vi "AddControlClass.vi"(4 "class":string, 5 "name":string, 6 "error in":errorcluster, 9 "PythonConverter_GUI in":refnum<class "PythonConverter_GUI.lvclass">) -> (0 "error out":errorcluster, 3 "PythonConverter_GUI out":refnum<class "PythonConverter_GUI.lvclass">)   [LabVIEW 2014, in "Raspberry Pi Compatible Compiler for LabVIEW.lvlib" / "PythonConverter_GUI.lvclass"]
uses:
  PythonConverter_GUI.lvclass
  PythonConverter_GUI.lvclass/PythonConverter_GUI.ctl
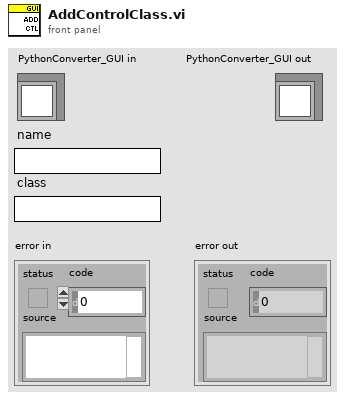
[diagram p1: front panel]
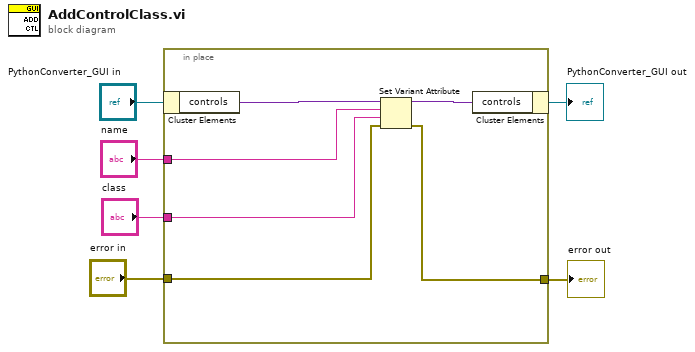
[diagram p0: block diagram]
diagram:
  n1 = in-place {
    in-place-border: "error in" -> [w10]
    in-place-border: [w9] -> w4
    in-place-border: "name" -> [w8]
    in-place-border: "class" -> [w7]
    n2 = in-place-cluster #1("PythonConverter_GUI in") -> ("controls"=w12:variant)
    n3 = Set Variant Attribute(Variant=w12, name=w8, value=w7, error in=w10) -> (Variant out=w11:variant, error out=w9:errorcluster)  [unwired: 1 out]
    n4 = in-place-cluster #1("controls"=w11) -> (→"PythonConverter_GUI out":refnum<class "PythonConverter_GUI.lvclass">)
  }
  "error out" <- w4
